vi "Initialize.vi"(8 "error in (no error)":errorcluster, 10 "Info":T1, 11 "Image in":refnum<class "SVGImage.lvclass">) -> (0 "error out":errorcluster, 3 "Image out":refnum<class "SVGImage.lvclass">)   [LabVIEW 2019, in "SVGImage.lvclass"]
uses:
  SVGImage.lvclass
  C:/Users/Albro/Documents/GitHub/AFM-Lithography/lvsrc/Classes/Parse/SVG Object/SVG Object.lvclass
  InitializationInfo.ctl
  SVGImage.lvclass/SVGImage.ctl
  Write X.vi
  Write Y.vi
  Write Width.vi
  Write Height.vi
  Write Path.vi
  <vilib>/LabVIEW Open Source Project/OpenURI/openURI.lvlib
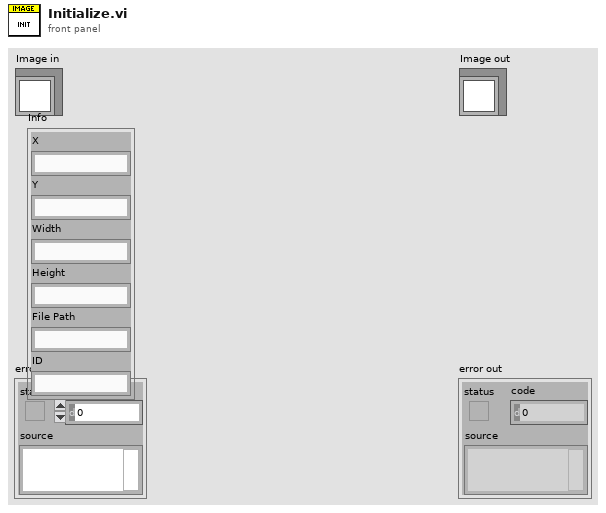
[diagram p1: front panel]
types:
  T1 = typedef "SVGImage.lvclass/InitializationInfo.ctl" = cluster{"X":string, "Y":string, "Width":string, "Height":string, "File Path":string, "ID":string}
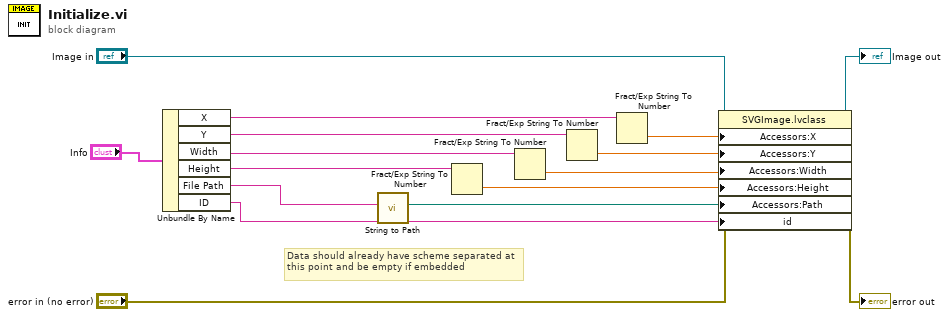
[diagram p0: block diagram]
diagram:
  # "Data should already have scheme separated at this point and be empty if embedded"
  n1 = Unbundle By Name("Info") -> ("X"=w13:string, "Y"=w12:string, "Width"=w11:string, "Height"=w10:string, "File Path"=w2:string, "ID"=w1:string)
  n2 = call <vilib>:"String to Path.vi"("common path"=w2) -> ("Path"=w3:path)  [unwired: 10 in]
  n3 = Fract/Exp String To Number(string=w10) -> (number=w6:dbl)  [unwired: 3 in, 1 out]
  n4 = Fract/Exp String To Number(string=w11) -> (number=w7:dbl)  [unwired: 3 in, 1 out]
  n5 = Fract/Exp String To Number(string=w12) -> (number=w8:dbl)  [unwired: 3 in, 1 out]
  n6 = Fract/Exp String To Number(string=w13) -> (number=w9:dbl)  [unwired: 3 in, 1 out]
  n7 = property class="SVGImage.lvclass"(reference="Image in", error in="error in (no error)", "Accessors:X"=w9, "Accessors:Y"=w8, "Accessors:Width"=w7, "Accessors:Height"=w6, "Accessors:Path"=w3, "id"=w1) -> (reference out=→"Image out":refnum<class "SVGImage.lvclass">, error out=→"error out":errorcluster)
